vi "logicaBotons.vi"(1 "Start IN's":T2, 2 "Entrada estat":enum16{"WAIT", "READ", ""}(ring), 3 "Power OFF IN's":T3) -> (0 "Cluster":T1)   [LabVIEW 2018]
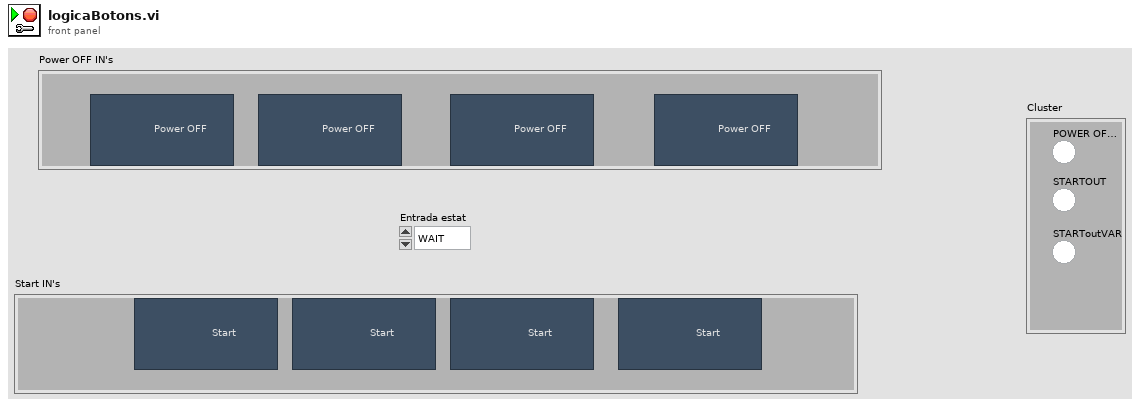
[diagram p1: front panel]
types:
  T1 = cluster{"POWER OFF OUT":bool, "STARTOUT":bool, "STARToutVAR":bool}
  T2 = cluster{"START 5":bool, "START 2":bool, "START 3":bool, "START 4":bool}
  T3 = cluster{"STOP":bool, "STOP 2":bool, "STOP 3":bool, "STOP 4":bool}
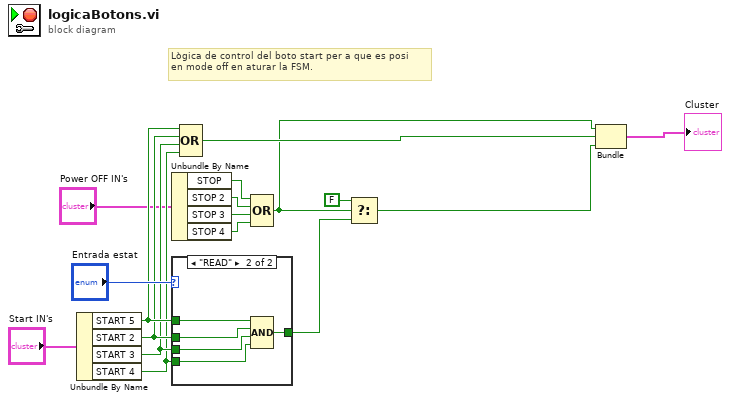
[diagram p0: block diagram]
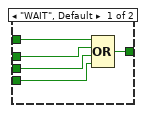
[diagram p2: hidden frame]
diagram:
  # "Lògica de control del boto start per a que es posi \nen mode off en aturar la FSM."
  n1 = Unbundle By Name("Start IN's") -> ("START 5"=w13:bool, "START 2"=w12:bool, "START 3"=w11:bool, "START 4"=w10:bool)
  n2 = Unbundle By Name("Power OFF IN's") -> ("STOP"=w8:bool, "STOP 2"=w7:bool, "STOP 3"=w6:bool, "STOP 4"=w5:bool)
  n3 = case shown="\"READ\"" "Entrada estat" {
    tunnel: w13 -> [w19 w27]
    tunnel: w12 -> [w22 w26]
    tunnel: w11 -> [w21 w25]
    tunnel: w10 -> [w20 w24]
    tunnel: [w18 w23] -> w16
    frame "WAIT", Default {
      n4 = Compound Arithmetic op=OR(w19, w22, w21, w20) -> (w18:bool)
    }
    frame "READ" {
      n5 = Compound Arithmetic op=AND(w27, w26, w25, w24) -> (w23:bool)
    }
  }
  n6 = Compound Arithmetic op=OR(w13, w12, w11, w10) -> (w3:bool)
  n7 = Compound Arithmetic op=OR(w8, w7, w6, w5) -> (w2:bool)
  n8 = Select(t=FALSE, s=w2, f=w16) -> (s? t:f=w1:bool)
  n9 = Bundle(w2, w3, "t"=w1) -> (→"Cluster":cluster{bool, bool, "t":bool})  [unwired: 1 in]
